vi "Evaluate Part 1.vi"(11 "Input":string="Time:      7  15   30\nDistance:  9  40  200") -> ()   [LabVIEW 2021]
uses:
  Race/Race.lvclass
panel:
  out "product":u64=288
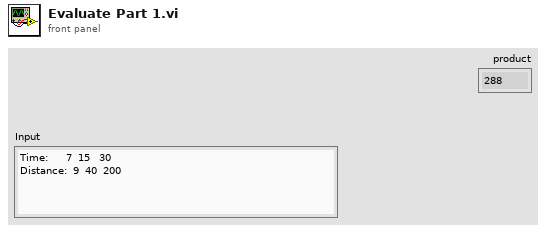
[diagram p1: front panel]
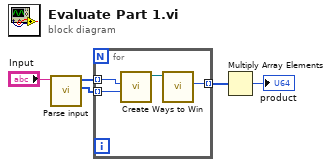
[diagram p0: block diagram]
diagram:
  n1 = call "Parse input.vi"("Input"="Input") -> ("Distances"=w3:u64[], "Times"=w4:u64[])  [unwired: 9 in]
  n2 = for {
    tunnel: w4 -> [w9] mode=indexing
    tunnel: w3 -> [w8] mode=indexing
    tunnel: [w6] -> w2 mode=indexing
    n3 = call "Create.vi"("Distance"=w8, "Time"=w9) -> ("Race Out"=w7:refnum<class "Race.lvclass">)  [unwired: 8 in, 1 out]
    n4 = call "Ways to Win.vi"("Race In"=w7) -> ("Ways to win"=w6:u64)  [unwired: 9 in, 1 out]
  }
  n5 = Multiply Array Elements(1:w2) -> (0:→"product":u64)
